vi "Autonomous Independent.vi"   [LabVIEW 2023]
doc: "This VI is called when autonomous begins, and will automatically be terminated when autonomous ends. You can carry out timed or sensor driven robot movement independently without needing to return to the caller."
uses:
  <vilib>/Rock Robotics/Network Tables/NT Read String.vi
panel:
  # "Be sure to right-click and choose Data Operations>>Make Current Value default if you want to save the array values with the VI"
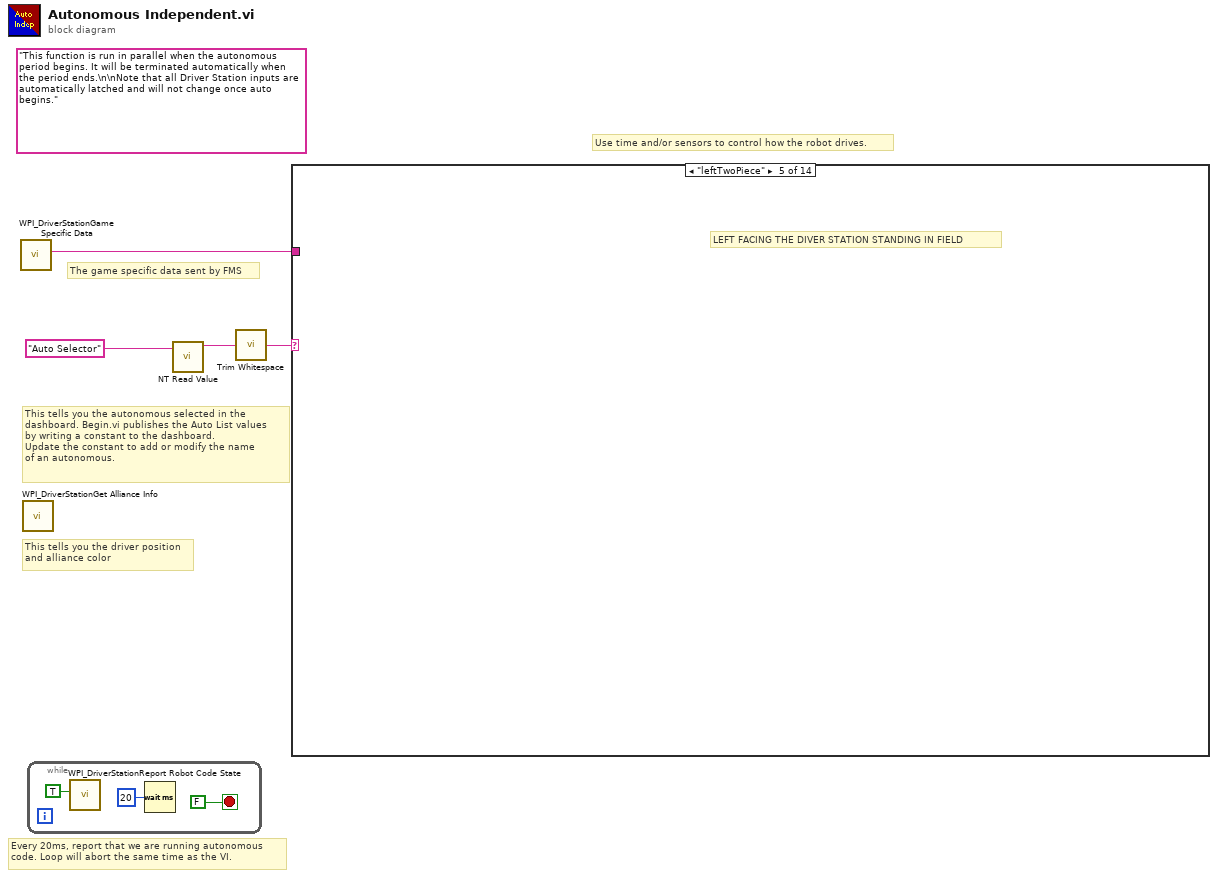
[diagram p0: block diagram]
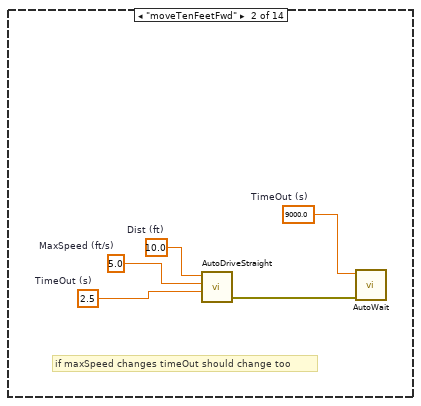
[diagram p3: hidden frame]
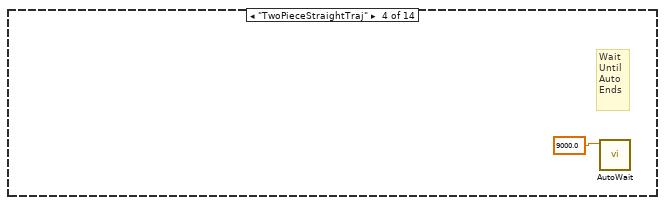
[diagram p5: hidden frame]
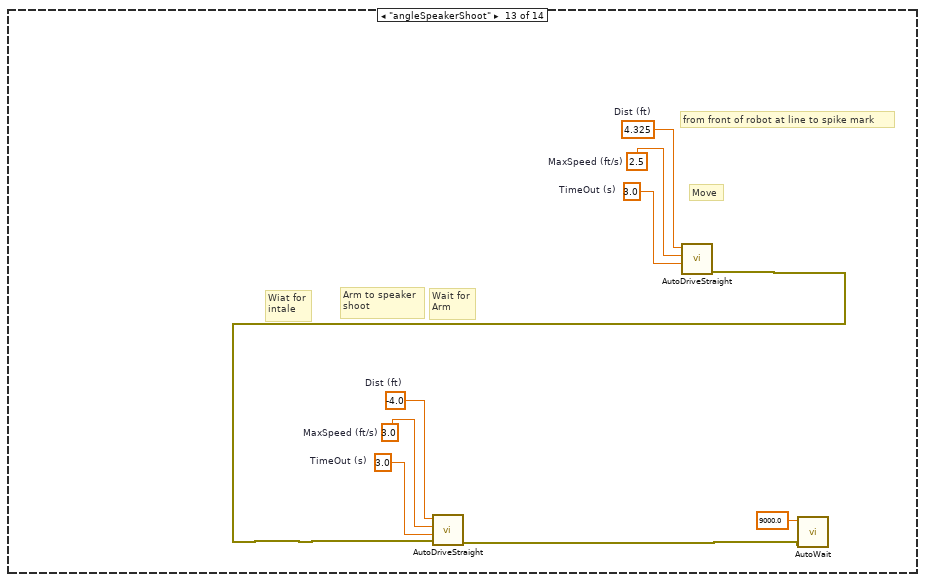
[diagram p13: hidden frame]
diagram:
  (unwired) "This function is run in parallel when the autonomous period begins. It will be terminated automatically when the period ends.\n\nNote that all Driver Station inputs are automatically latched and will not change once auto begins."
  # "The game specific data sent by FMS"
  # "This tells you the autonomous selected in the \ndashboard. Begin.vi publishes the Auto List values\nby writing a constant to the dashboard.\nUpdate the constant to add or modify the name\nof an autonomous."
  # "Every 20ms, report that we are running autonomous\ncode. Loop will abort the same time as the VI."
  # "Use time and/or sensors to control how the robot drives."
  # "This tells you the driver position\nand alliance color"
  n1 = call <vilib>:"WPI_DriverStationGame Specific Data.vi"() -> ("Game Specific Data"=w3:string)  [unwired: 11 in]
  n2 = call <vilib>:"WPI_DriverStationGet Alliance Info.vi"() -> ()  [unwired: 12 out]
  n3 = while {
    stop <- FALSE stop-if-true
    n4 = call <vilib>:"WPI_DriverStationReport Robot Code State.vi"("Autonomous"=TRUE) -> ()  [unwired: 10 in, 1 out]
    n5 = Wait (ms)(milliseconds to wait=u32 20) -> ()  [unwired: 1 out]
  }
  n6 = call-poly <vilib>:"NT Read Value.vi"("name"="Auto Selector" ("Name")) -> ("value"=w1:string)  [unwired: 8 in, 2 out]
  n7 = call <vilib>:"Trim Whitespace.vi"("string"=w1) -> ("trimmed string"=w2:string)  [unwired: 1 in]
  n8 = case shown="\"leftTwoPiece\"" w2 {
    tunnel: w3 -> [_ _ _ _ _ _ _ _ _ _ _ _ _ _]
    frame Default {
      # "You can put your main auto here, or you can right-click on the case and make any\nother frame be the default case."
      # "This is the frame that will execute if no selection is made, or if it is not recognized"
    }
    frame "moveTenFeetFwd" {
      w8 = 9000.0  # TimeOut (s)
      w10 = 2.5  # TimeOut (s)
      w11 = 5.0  # MaxSpeed (ft/s)
      w12 = 10.0  # Dist (ft)
      # "if maxSpeed changes timeOut should change too"
      n9 = call "AutoDriveStraight.vi"("TimeOut (s)"=w10, "MaxSpeed (ft/s)"=w11, "Dist (ft)"=w12) -> ("error out"=w9:errorcluster)  [unwired: 8 in]
      n10 = call "AutoWait.vi"("error in (no error)"=w9, "TimeOut (s)"=w8) -> ()  [unwired: 9 in, 1 out]
    }
    frame "twoPieceStraight" {
    }
    frame "TwoPieceStraightTraj" {
      # "Wait\nUntil\nAuto \nEnds"
      n11 = call "AutoWait.vi"("TimeOut (s)"=9000.0) -> ()  [unwired: 10 in, 1 out]
    }
    frame "leftTwoPiece" {
      # "LEFT FACING THE DIVER STATION STANDING IN FIELD"
    }
    frame "BLUELeftTwoPiece" {
      # "LEFT FACING FIELD FROM DRIVERS STATION"
    }
    frame "rightTwoPiece" {
      # "RIGHT FACING THE DIVER STATION STANDING IN FIELD"
    }
    frame "BLUERIghtTwoPiece" {
      # "RIGHT FACING FIELD FROM DRIVERS STATION"
    }
    frame "Straight2PieceThenLeftNoteTraj" {
    }
    frame "BlueStraight2PieceThenLeftNoteTraj" {
    }
    frame "TwoPiecestraightThenCenterLineTraj" {
    }
    frame "BlueTwoPiecestraightThenCenterLineTraj" {
    }
    frame "angleSpeakerShoot" {
      w16 = 3.0  # TimeOut (s)
      w17 = 3.0  # MaxSpeed (ft/s)
      w18 = -4.0  # Dist (ft)
      w20 = 3.0  # TimeOut (s)
      w21 = 2.5  # MaxSpeed (ft/s)
      w22 = 4.325  # Dist (ft)
      # "Wait for\nArm"
      # "Arm to speaker\nshoot"
      # "Wiat for\nintale"
      # "Move"
      # "from front of robot at line to spike mark"
      n12 = call "AutoDriveStraight.vi"("TimeOut (s)"=w20, "MaxSpeed (ft/s)"=w21, "Dist (ft)"=w22) -> ("error out"=w15:errorcluster)  [unwired: 8 in]
      n13 = call "AutoDriveStraight.vi"("error in (no error)"=w15, "TimeOut (s)"=w16, "MaxSpeed (ft/s)"=w17, "Dist (ft)"=w18) -> ("error out"=w14:errorcluster)  [unwired: 7 in]
      n14 = call "AutoWait.vi"("error in (no error)"=w14, "TimeOut (s)"=9000.0) -> ()  [unwired: 9 in, 1 out]
    }
    frame "Your Turn" {
    }
  }
